vi "2DInterpPerfData.vi"() -> ()   [LabVIEW 2018]
uses:
  <vilib>/Platform/TimedLoop/XDataNode/timing_clust.ctl
  <vilib>/Platform/TimedLoop/XDataNode/nitl_modes.ctl
  <vilib>/Platform/TimedLoop/XDataNode/wakeup.ctl
  <vilib>/Utility/file.llb/Read Delimited Spreadsheet (DBL).vi
  <vilib>/gmath/interp.llb/Interpolate 2D (1d xi,yi).vi
  <vilib>/platform/TimedLoop/XDataNode/XDataNode.xnode
  <vilib>/Platform/TimedLoop/XDataNode/XDNodeRunTimeDep.lvlib
  <vilib>/gmath/NI_Gmath.lvlib
panel:
  in  "stop":bool
  in  "ntimes":i32=1
  out "Error":errorcluster
  in  "yi":dbl[](array[numeric])
  in  "xi":dbl[](array[numeric])
  out "yi used":dbl[][](array[numeric])
  out "xi used":dbl[][](array[numeric])
  out "error":i32
  out "zi":dbl[][](array[numeric])
  out "cp":dbl[][](array[numeric])
  out "pitch":dbl[](array[numeric])
  out "tsr":dbl[](array[numeric])
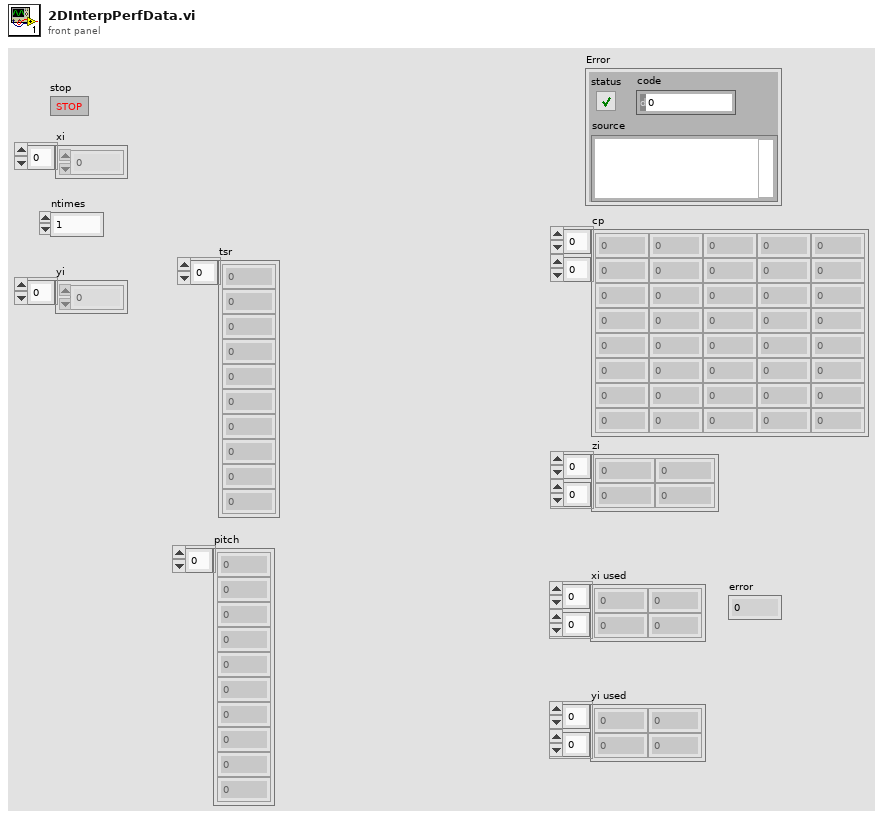
[diagram p1: front panel]
types:
  T1 = typedef "XDNodeRunTimeDep.lvlib/timing_clust.ctl" = cluster{"Expected End [f-1]":u64, "Actual End [f-1]":u64, "Finished Late? [f-1]":bool, "Expected End [i-1]":u64, "Actual End [i-1]":u64, "Finished Late? [i-1]":bool, "Expected Start [i]":u64, "Actual Start [i]":u64, "Expected Start [f]":u64, "Actual Start [f]":u64, "Source Name":string, "Structure Name":string, "Period":i64, "Deadline":i64, "Offset":i64, "Start":i64, "Priority":i32, "Timeout":i32, "Mode":T2, "Wakeup Reason":T3, "Error":errorcluster, "Source Type":string, "Secondary Source Type":string, "Global End Time":u64, "Global Start Time":u64, "Frame Duration":u64, "Iteration Duration":u64, "Assigned CPU":i32, "I/O Scan Engine Mode":u32}
  T2 = typedef "XDNodeRunTimeDep.lvlib/nitl_modes.ctl" = enum32{"No Change", "Process missed periods, maintain original phase", "Discard missed periods, maintain original phase", "Process missed periods, ignore original phase", "Discard missed periods, ignore original phase"}
  T3 = typedef "XDNodeRunTimeDep.lvlib/wakeup.ctl" = enum32{"Normal", "Aborted", "Asynchronous wakeup", "Timing source error", "Timed loop error", "Timeout"}
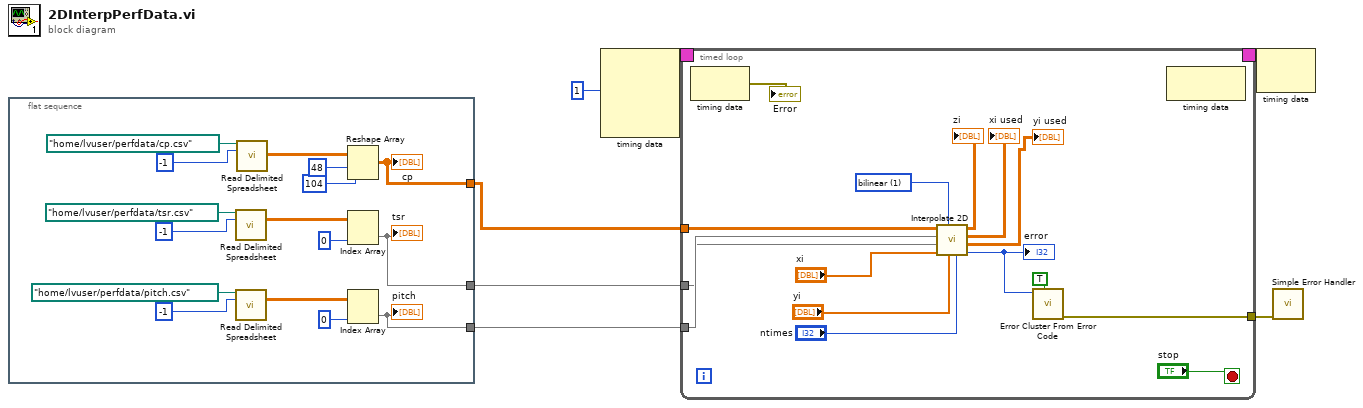
[diagram p0: block diagram]
diagram:
  n1 = flat-sequence {
    tunnel: [w10] -> w4
    tunnel: [w9] -> w3
    tunnel: [w8] -> w2
    frame #0 {
      n2 = call-poly <vilib>:"Read Delimited Spreadsheet.vi"("file path (dialog if empty)"=path "/home/lvuser/perfdata/tsr.csv", "number of rows (all:-1)"=-1) -> ("all rows"=w17:dbl[][])  [unwired: 8 in, 5 out]
      n3 = call-poly <vilib>:"Read Delimited Spreadsheet.vi"("file path (dialog if empty)"=path "/home/lvuser/perfdata/pitch.csv", "number of rows (all:-1)"=-1) -> ("all rows"=w14:dbl[][])  [unwired: 8 in, 5 out]
      n4 = call-poly <vilib>:"Read Delimited Spreadsheet.vi"("file path (dialog if empty)"=path "/home/lvuser/perfdata/cp.csv", "number of rows (all:-1)"=-1) -> ("all rows"=w13:dbl[][])  [unwired: 8 in, 5 out]
      n5 = Reshape Array(w13, 48 ("dimension size"), 104 ("dimension size")) -> (w8:dbl[][])
      "cp" <- w8
      n6 = Index Array(array=w17, index (col)=0 ("disabled index (col)")) -> (element=w10:dbl[])  [unwired: 1 in]
      "tsr" <- w10
      n7 = Index Array(array=w14, index (col)=0 ("disabled index (col)")) -> (element=w9:dbl[])  [unwired: 1 in]
      "pitch" <- w9
    }
  }
  n8 = node-c288(i64 1 ("Period")) -> (w7:T1)  [unwired: 3 in]
  n9 = timed-loop {
    timing: w7 -> [_]
    timing-out: [_] -> w6
    tunnel: w4 -> [w24]
    tunnel: w3 -> [w25]
    tunnel: w2 -> [w37]
    tunnel: [w34] -> w1
    stop <- "stop" stop-if-true
    w38 = 1 items=["nearest", "bilinear", "bicubic", "bicubic spline"] ("method")
    n10 = node-c288() -> (→"Error":errorcluster)  [unwired: 1 in]
    n11 = call-poly <vilib>:"Interpolate 2D.vi"("ntimes"="ntimes", "yi"="yi", "method"=w38, "xi"="xi", "Y"=w24, "X"=w25, "Z"=w37) -> ("error"=w35:i32, "yi used"=→"yi used":dbl[][], "xi used"=→"xi used":dbl[][], "zi"=→"zi":dbl[][])  [unwired: 1 in]
    "error" <- w35
    n12 = call <vilib>:"Error Cluster From Error Code.vi"("show call chain? (False)"=TRUE, "error code (0)"=w35) -> ("error out"=w34:errorcluster)  [unwired: 7 in]
    n13 = node-c288() -> ()  [unwired: 1 in, 1 out]
  }
  n14 = node-c288(w6) -> ()  [unwired: 1 out]
  n15 = call <vilib>:"Simple Error Handler.vi"("error in (no error)"=w1) -> ()  [unwired: 4 in, 5 out]
